vi "filter.get.state.vi"(11 "filter.data in":T1 {"get.state"."v"."Quantity" format="%.0x"; "get.state"."v"."OrderId" format="%.0x"; "mem.cmd"."ord.2"."v"."Quantity" format="%016x"; "mem.cmd"."ord.2"."v"."OrderId" format="%016x"; "mem.cmd"."ord.1"."v"."Quantity" format="%016x"; "mem.cmd"."ord.1"."v"."OrderId" format="%016x"; "mem.cmd"."ticker"."v"."Symbol" format="%016x"; "mem.cmd"."order.slot.value"."Quantity" format="%016x"; "mem.cmd"."order.slot.value"."OrderId" format="%016x"; "debug"."v"."slot.3" format="%.0x"; "debug"."v"."slot.2" format="%.0x"; "debug"."v"."slot.1" format="%.0x"; "debug"."v"."slot.0" format="%.0x"; "Scratch"."OrderId" format="%016x"; "hash.2"."data.in" format="%.0x"; "hash.2"."crc32.out" format="%.0x"; "hash.1"."data.in" format="%.0x"; "hash.1"."crc32.out" format="%.0x"}) -> (3 "filter.data out":T1 {"get.state"."v"."Quantity" format="%.0x"; "get.state"."v"."OrderId" format="%.0x"; "mem.cmd"."ord.2"."v"."Quantity" format="%016x"; "mem.cmd"."ord.2"."v"."OrderId" format="%016x"; "mem.cmd"."ord.1"."v"."Quantity" format="%016x"; "mem.cmd"."ord.1"."v"."OrderId" format="%016x"; "mem.cmd"."ticker"."v"."Symbol" format="%016x"; "mem.cmd"."order.slot.value"."Quantity" format="%016x"; "mem.cmd"."order.slot.value"."OrderId" format="%016x"; "debug"."v"."slot.3" format="%.0x"; "debug"."v"."slot.2" format="%.0x"; "debug"."v"."slot.1" format="%.0x"; "debug"."v"."slot.0" format="%.0x"; "Scratch"."OrderId" format="%016x"; "hash.2"."data.in" format="%.0x"; "hash.2"."crc32.out" format="%.0x"; "hash.1"."data.in" format="%.0x"; "hash.1"."crc32.out" format="%.0x"})   [LabVIEW 2020]
uses:
  order.slot.ctl
  ticker.slot.ctl
  filter.memory.command.ctl
  filter.states.ctl
  filter.state.slot.ctl
  filter.state.ctl
  order.slot.hm.ctl
  order.slot.access.ctl
  ticker.slot.access.ctl
  filter.debug.slot.ctl
  filter.debug.ctl
  filter.data.scratch.ctl
  Market.Data.Common/fpga/orderbook.command.ctl
  Market.Data.Common/fpga/fpganow.common.fpga.lvlib
  filter.data.ctl
  Market.Data.Common/fpga/orderbook.command.type.ctl
  filter.hash.ctl
  Filter.lvclass
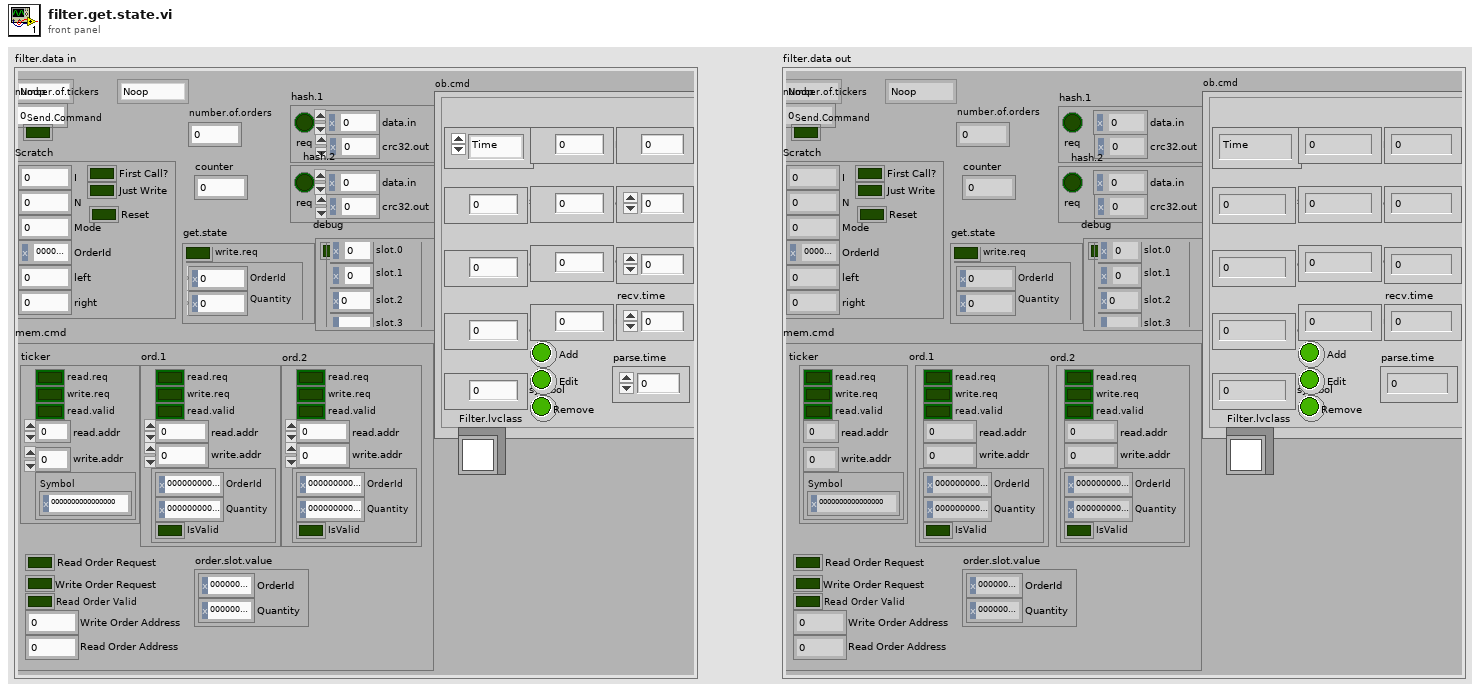
[diagram p1: front panel]
types:
  T1 = typedef "filter.data.ctl" = cluster{"filter.state":T2, "number.of.tickers":u32, "filter.saved.state":T2, "Send.Command":bool, "hash.1":T3, "hash.2":T3, "Scratch":T4, "debug":T5, "mem.cmd":T7, "get.state":T13, "ob.cmd":T15, "number.of.orders":u32, "Filter.lvclass":refnum<class "Filter.lvclass">, "counter":i16}
  T2 = typedef "filter.states.ctl" = enum16{"Noop", "Reset", "Debug", "Configuration", "Wait.for.Command", "Filter.Add", "Filter.Other", "Insert.Order", "Delete Order", "Get.State", "Get.Watchlist", "Get.Memory"}
  T3 = typedef "filter.hash.ctl" = cluster{"req":bool, "data.in":u64, "crc32.out":u32}
  T4 = typedef "filter.data.scratch.ctl" = cluster{"I":u32, "N":u32, "Mode":u32, "OrderId":u64, "First Call?":bool, "Just Write":bool, "left":u32, "right":u32, "Reset":bool}
  T5 = typedef "filter.debug.ctl" = cluster{"write":bool, "v":T6}
  T6 = typedef "filter.debug.slot.ctl" = cluster{"slot.0":u64, "slot.1":u64, "slot.2":u64, "slot.3":u64}
  T7 = typedef "filter.memory.command.ctl" = cluster{"Read Order Request":bool, "Write Order Request":bool, "Read Order Valid":bool, "Write Order Address":u32, "Read Order Address":u32, "order.slot.value":T8, "ticker":T9, "ord.1":T11, "ord.2":T11}
  T8 = typedef "order.slot.ctl" = cluster{"OrderId":u64, "Quantity":u64}
  T9 = typedef "ticker.slot.access.ctl" = cluster{"read.req":bool, "write.req":bool, "read.valid":bool, "read.addr":u32, "write.addr":u32, "v":T10}
  T10 = typedef "ticker.slot.ctl" = cluster{"Symbol":u64}
  T11 = typedef "order.slot.access.ctl" = cluster{"read.req":bool, "write.req":bool, "read.valid":bool, "read.addr":u32, "write.addr":u32, "v":T12}
  T12 = typedef "order.slot.hm.ctl" = cluster{"OrderId":u64, "Quantity":u64, "IsValid":bool}
  T13 = typedef "filter.state.ctl" = cluster{"write.req":bool, "v":T14}
  T14 = typedef "filter.state.slot.ctl" = cluster{"OrderId":u64, "Quantity":u64}
  T15 = typedef "fpganow.common.fpga.lvlib/orderbook.command.ctl" = cluster{"type":T16, "side":u8, "orderId ":u64, "quantity":u32, "symbol":u64, "price":u64, "executed.qty":u32, "canceled.qty":u32, "remaining.qty":u32, "seconds":u64, "nanoseconds":u64, "Add":bool, "Edit":bool, "Remove":bool, "seq no":u32, "recv.time":u64, "parse.time":u64}
  T16 = typedef "fpganow.common.fpga.lvlib/orderbook.command.type.ctl" = enum8{"Time", "AddOrder", "OrderExecuted", "OrderExecutedAtPrice", "ReduceSize", "ModifyOrder", "DeleteOrder", "Get.Everything", "Get.All.Orders", "Get.Top"}
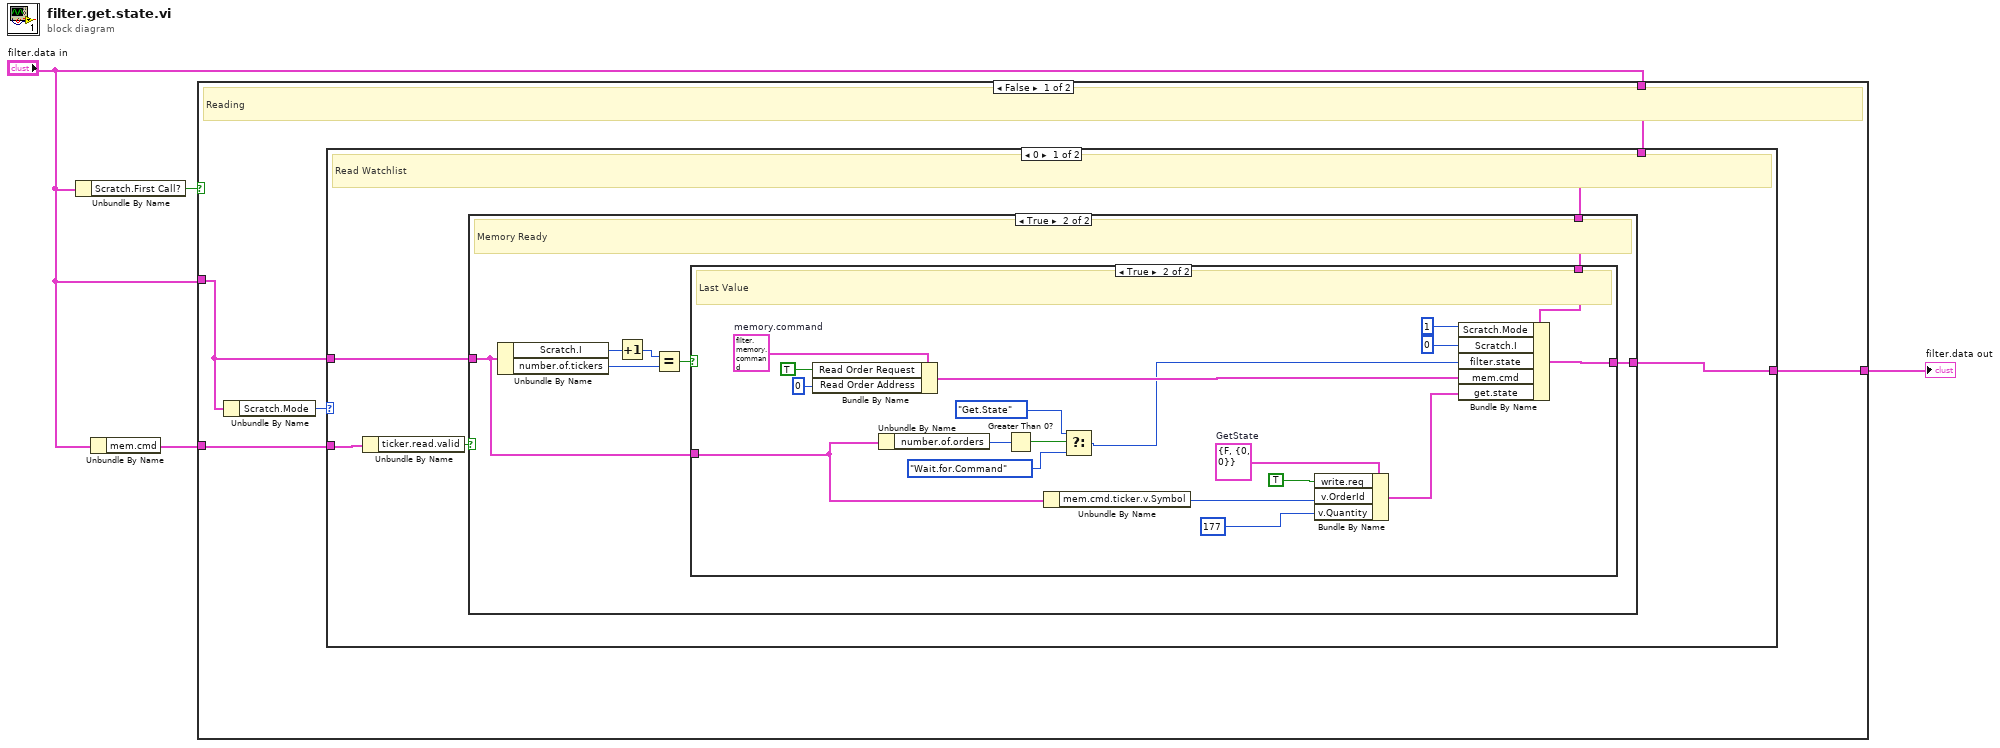
[diagram p0: block diagram]
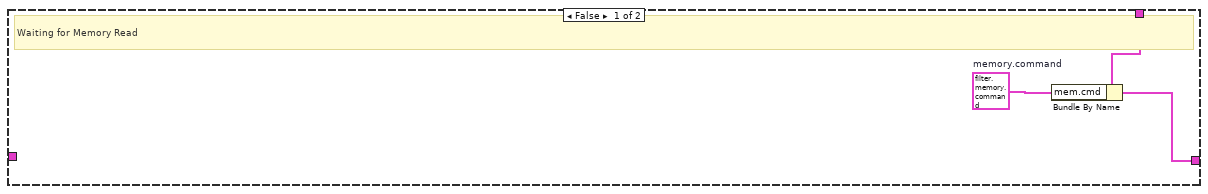
[diagram p2: hidden frame]
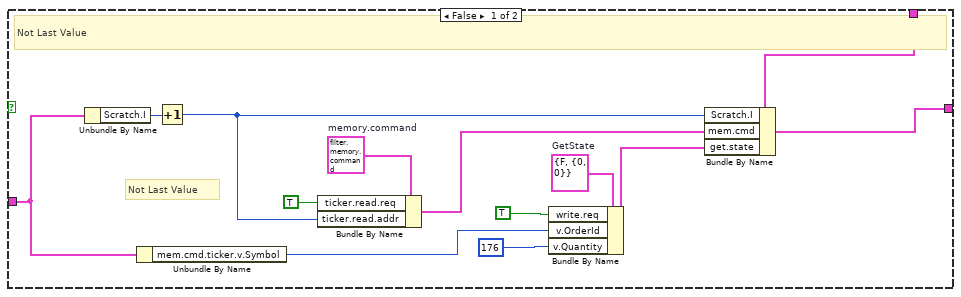
[diagram p3: hidden frame]
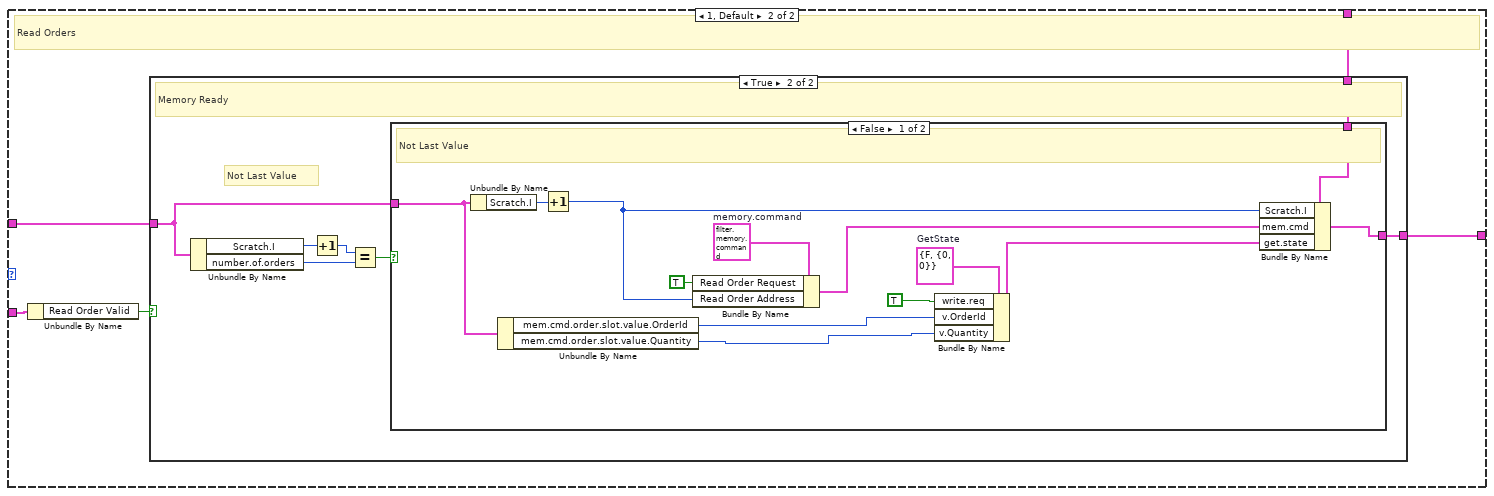
[diagram p4: hidden frame]
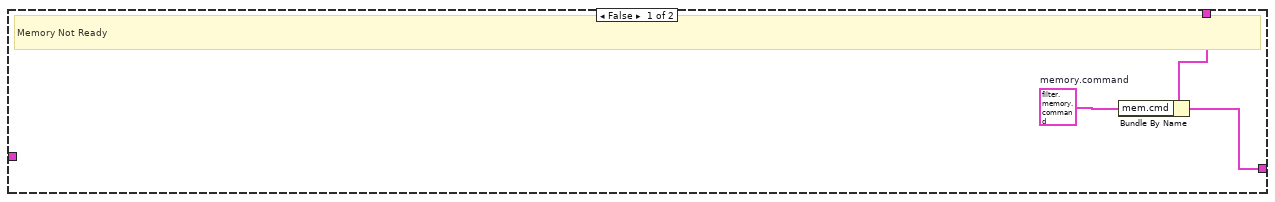
[diagram p5: hidden frame]
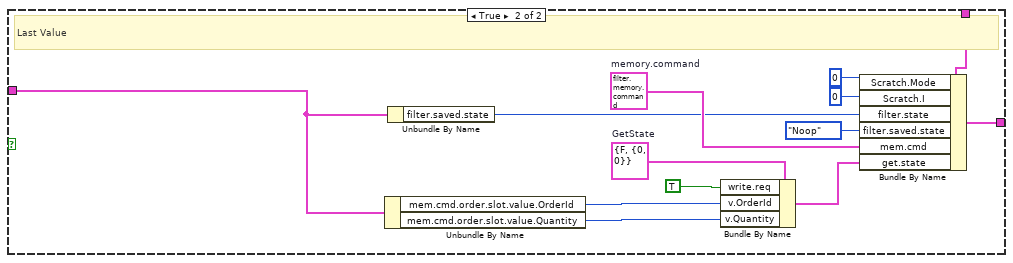
[diagram p6: hidden frame]
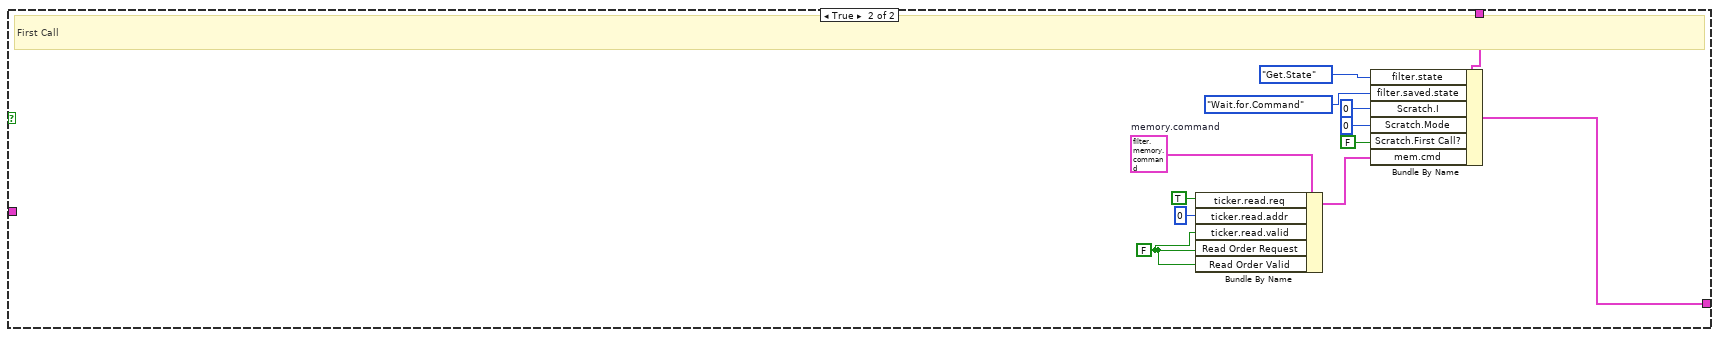
[diagram p7: hidden frame]
diagram:
  n1 = Unbundle By Name("filter.data in") -> ("Scratch.First Call?"=w1:bool)
  n2 = Unbundle By Name("filter.data in") -> ("mem.cmd"=w4:T7)
  n3 = case shown="False" w1 {
    tunnel: "filter.data in" -> [w8 w109]
    tunnel: [w9 w108] -> w2
    tunnel: "filter.data in" -> [w6 _]
    tunnel: w4 -> [w7 _]
    frame False {
      # "Reading"
      n4 = Unbundle By Name(w6) -> ("Scratch.Mode"=w5:u32)
      n5 = case shown="0" w5 {
        tunnel: [w14 w61] -> w9
        tunnel: w8 -> [w13 w60]
        tunnel: w7 -> [w11 w58]
        tunnel: w6 -> [w10 w57]
        frame 0 {
          # "Read Watchlist"
          n6 = Unbundle By Name(w11) -> ("ticker.read.valid"=w12:bool)
          n7 = case shown="True" w12 {
            tunnel: [w15 w18] -> w14
            tunnel: w13 -> [w17 w19]
            tunnel: w10 -> [_ w20]
            frame False {
              w16 = T7 {"Read Order Request"=FALSE, "Write Order Request"=FALSE, "Read Order Valid"=FALSE, "Write Order Address"=0, "Read Order Address"=0, "order.slot.value"={"OrderId"=0, "Quantity"=0}, "ticker"={"read.req"=FALSE, "write.req"=FALSE, "read.valid"=FALSE, "read.addr"=0, "write.addr"=0, "v"={"Symbol"=0}}, "ord.1"={"read.req"=FALSE, "write.req"=FALSE, "read.valid"=FALSE, "read.addr"=0, "write.addr"=0, "v"={"OrderId"=0, "Quantity"=0, "IsValid"=FALSE}}, "ord.2"={"read.req"=FALSE, "write.req"=FALSE, "read.valid"=FALSE, "read.addr"=0, "write.addr"=0, "v"={"OrderId"=0, "Quantity"=0, "IsValid"=FALSE}}}  # memory.command
              # "Waiting for Memory Read"
              n8 = Bundle By Name(cluster=w17, "mem.cmd"=w16) -> (w15:T1)
            }
            frame True {
              # "Memory Ready"
              n9 = Unbundle By Name(w20) -> ("Scratch.I"=w24:u32, "number.of.tickers"=w22:u32)
              n10 = Increment(x=w24) -> (x+1=w23:u32)
              n11 = Equal?(x=w23, y=w22) -> (x = y?=w21:bool)
              n12 = case shown="True" w21 {
                tunnel: w20 -> [w30 w43]
                tunnel: w19 -> [w26 w56]
                tunnel: [w37 w55] -> w18
                frame False {
                  w33 = T13 {"write.req"=FALSE, "v"={"OrderId"=0, "Quantity"=0}}  # GetState
                  w36 = T7 {"Read Order Request"=FALSE, "Write Order Request"=FALSE, "Read Order Valid"=FALSE, "Write Order Address"=0, "Read Order Address"=0, "order.slot.value"={"OrderId"=0, "Quantity"=0}, "ticker"={"read.req"=FALSE, "write.req"=FALSE, "read.valid"=FALSE, "read.addr"=0, "write.addr"=0, "v"={"Symbol"=0}}, "ord.1"={"read.req"=FALSE, "write.req"=FALSE, "read.valid"=FALSE, "read.addr"=0, "write.addr"=0, "v"={"OrderId"=0, "Quantity"=0, "IsValid"=FALSE}}, "ord.2"={"read.req"=FALSE, "write.req"=FALSE, "read.valid"=FALSE, "read.addr"=0, "write.addr"=0, "v"={"OrderId"=0, "Quantity"=0, "IsValid"=FALSE}}}  # memory.command
                  # "Not Last Value"
                  # "Not Last Value"
                  n13 = Unbundle By Name(w30) -> ("Scratch.I"=w34:u32)
                  n14 = Unbundle By Name(w30) -> ("mem.cmd.ticker.v.Symbol"=w29:u64)
                  n15 = Increment(x=w34) -> (x+1=w27:u32)
                  n16 = Bundle By Name(cluster=w36, "ticker.read.req"=TRUE ("Read.Request"), "ticker.read.addr"=w27) -> (w35:T7)
                  n17 = Bundle By Name(cluster=w33, "write.req"=TRUE ("Write.to.Debug"), "v.OrderId"=w29, "v.Quantity"=u64 176 ("debug.slot.OrderId")) -> (w32:T13)
                  n18 = Bundle By Name(cluster=w26, "Scratch.I"=w27, "mem.cmd"=w35, "get.state"=w32) -> (w37:T1)
                }
                frame True {
                  w44 = T13 {"write.req"=FALSE, "v"={"OrderId"=0, "Quantity"=0}}  # GetState
                  w48 = T7 {"Read Order Request"=FALSE, "Write Order Request"=FALSE, "Read Order Valid"=FALSE, "Write Order Address"=0, "Read Order Address"=0, "order.slot.value"={"OrderId"=0, "Quantity"=0}, "ticker"={"read.req"=FALSE, "write.req"=FALSE, "read.valid"=FALSE, "read.addr"=0, "write.addr"=0, "v"={"Symbol"=0}}, "ord.1"={"read.req"=FALSE, "write.req"=FALSE, "read.valid"=FALSE, "read.addr"=0, "write.addr"=0, "v"={"OrderId"=0, "Quantity"=0, "IsValid"=FALSE}}, "ord.2"={"read.req"=FALSE, "write.req"=FALSE, "read.valid"=FALSE, "read.addr"=0, "write.addr"=0, "v"={"OrderId"=0, "Quantity"=0, "IsValid"=FALSE}}}  # memory.command
                  # "Last Value"
                  n19 = Bundle By Name(cluster=w48, "Read Order Request"=TRUE ("Read Order\nRequest"), "Read Order Address"=u32 0 ("Read Order\nAddress")) -> (w47:T7)
                  n20 = Unbundle By Name(w43) -> ("number.of.orders"=w42:u32)
                  n21 = Greater Than 0?(x=w42) -> (x > 0?=w41:bool)
                  n22 = Unbundle By Name(w43) -> ("mem.cmd.ticker.v.Symbol"=w52:u64)
                  n23 = Select(t=filter.states."Get.State" ("filter.state"), s=w41, f=filter.states."Wait.for.Command") -> (s? t:f=w39:T2)
                  n24 = Bundle By Name(cluster=w44, "write.req"=TRUE ("Write.to.Debug"), "v.OrderId"=w52, "v.Quantity"=u64 177 ("debug.slot.OrderId")) -> (w54:T13)
                  n25 = Bundle By Name(cluster=w56, "Scratch.Mode"=u32 1, "Scratch.I"=u32 0, "filter.state"=w39, "mem.cmd"=w47, "get.state"=w54) -> (w55:T1)
                }
              }
            }
          }
        }
        frame 1, Default {
          # "Read Orders"
          n26 = Unbundle By Name(w58) -> ("Read Order Valid"=w59:bool)
          n27 = case shown="True" w59 {
            tunnel: [w62 w65] -> w61
            tunnel: w60 -> [w64 w66]
            tunnel: w57 -> [_ w67]
            frame False {
              w63 = T7 {"Read Order Request"=FALSE, "Write Order Request"=FALSE, "Read Order Valid"=FALSE, "Write Order Address"=0, "Read Order Address"=0, "order.slot.value"={"OrderId"=0, "Quantity"=0}, "ticker"={"read.req"=FALSE, "write.req"=FALSE, "read.valid"=FALSE, "read.addr"=0, "write.addr"=0, "v"={"Symbol"=0}}, "ord.1"={"read.req"=FALSE, "write.req"=FALSE, "read.valid"=FALSE, "read.addr"=0, "write.addr"=0, "v"={"OrderId"=0, "Quantity"=0, "IsValid"=FALSE}}, "ord.2"={"read.req"=FALSE, "write.req"=FALSE, "read.valid"=FALSE, "read.addr"=0, "write.addr"=0, "v"={"OrderId"=0, "Quantity"=0, "IsValid"=FALSE}}}  # memory.command
              # "Memory Not Ready"
              n28 = Bundle By Name(cluster=w64, "mem.cmd"=w63) -> (w62:T1)
            }
            frame True {
              # "Not Last Value"
              # "Memory Ready"
              n29 = Unbundle By Name(w67) -> ("Scratch.I"=w71:u32, "number.of.orders"=w69:u32)
              n30 = Increment(x=w71) -> (x+1=w70:u32)
              n31 = Equal?(x=w70, y=w69) -> (x = y?=w68:bool)
              n32 = case shown="False" w68 {
                tunnel: w67 -> [w78 w93]
                tunnel: w66 -> [w76 w97]
                tunnel: [w84 w96] -> w65
                frame False {
                  w72 = T13 {"write.req"=FALSE, "v"={"OrderId"=0, "Quantity"=0}}  # GetState
                  w83 = T7 {"Read Order Request"=FALSE, "Write Order Request"=FALSE, "Read Order Valid"=FALSE, "Write Order Address"=0, "Read Order Address"=0, "order.slot.value"={"OrderId"=0, "Quantity"=0}, "ticker"={"read.req"=FALSE, "write.req"=FALSE, "read.valid"=FALSE, "read.addr"=0, "write.addr"=0, "v"={"Symbol"=0}}, "ord.1"={"read.req"=FALSE, "write.req"=FALSE, "read.valid"=FALSE, "read.addr"=0, "write.addr"=0, "v"={"OrderId"=0, "Quantity"=0, "IsValid"=FALSE}}, "ord.2"={"read.req"=FALSE, "write.req"=FALSE, "read.valid"=FALSE, "read.addr"=0, "write.addr"=0, "v"={"OrderId"=0, "Quantity"=0, "IsValid"=FALSE}}}  # memory.command
                  # "Not Last Value"
                  n33 = Unbundle By Name(w78) -> ("Scratch.I"=w81:u32)
                  n34 = Unbundle By Name(w78) -> ("mem.cmd.order.slot.value.OrderId"=w73:u64, "mem.cmd.order.slot.value.Quantity"=w74:u64)
                  n35 = Increment(x=w81) -> (x+1=w75:u32)
                  n36 = Bundle By Name(cluster=w83, "Read Order Request"=TRUE ("Read.Request"), "Read Order Address"=w75) -> (w82:T7)
                  n37 = Bundle By Name(cluster=w72, "write.req"=TRUE ("Write.to.Debug"), "v.OrderId"=w73, "v.Quantity"=w74) -> (w80:T13)
                  n38 = Bundle By Name(cluster=w76, "Scratch.I"=w75, "mem.cmd"=w82, "get.state"=w80) -> (w84:T1)
                }
                frame True {
                  w85 = T13 {"write.req"=FALSE, "v"={"OrderId"=0, "Quantity"=0}}  # GetState
                  w92 = T7 {"Read Order Request"=FALSE, "Write Order Request"=FALSE, "Read Order Valid"=FALSE, "Write Order Address"=0, "Read Order Address"=0, "order.slot.value"={"OrderId"=0, "Quantity"=0}, "ticker"={"read.req"=FALSE, "write.req"=FALSE, "read.valid"=FALSE, "read.addr"=0, "write.addr"=0, "v"={"Symbol"=0}}, "ord.1"={"read.req"=FALSE, "write.req"=FALSE, "read.valid"=FALSE, "read.addr"=0, "write.addr"=0, "v"={"OrderId"=0, "Quantity"=0, "IsValid"=FALSE}}, "ord.2"={"read.req"=FALSE, "write.req"=FALSE, "read.valid"=FALSE, "read.addr"=0, "write.addr"=0, "v"={"OrderId"=0, "Quantity"=0, "IsValid"=FALSE}}}  # memory.command
                  # "Last Value"
                  n39 = Unbundle By Name(w93) -> ("mem.cmd.order.slot.value.OrderId"=w87:u64, "mem.cmd.order.slot.value.Quantity"=w86:u64)
                  n40 = Unbundle By Name(w93) -> ("filter.saved.state"=w91:T2)
                  n41 = Bundle By Name(cluster=w85, "write.req"=TRUE ("Write.to.Debug"), "v.OrderId"=w87, "v.Quantity"=w86) -> (w95:T13)
                  n42 = Bundle By Name(cluster=w97, "Scratch.Mode"=u32 0, "Scratch.I"=u32 0, "filter.state"=w91, "filter.saved.state"=filter.states."Noop", "mem.cmd"=w92, "get.state"=w95) -> (w96:T1)
                }
              }
            }
          }
        }
      }
    }
    frame True {
      w99 = FALSE ("Read Ticker Valid")
      w104 = T7 {"Read Order Request"=FALSE, "Write Order Request"=FALSE, "Read Order Valid"=FALSE, "Write Order Address"=0, "Read Order Address"=0, "order.slot.value"={"OrderId"=0, "Quantity"=0}, "ticker"={"read.req"=FALSE, "write.req"=FALSE, "read.valid"=FALSE, "read.addr"=0, "write.addr"=0, "v"={"Symbol"=0}}, "ord.1"={"read.req"=FALSE, "write.req"=FALSE, "read.valid"=FALSE, "read.addr"=0, "write.addr"=0, "v"={"OrderId"=0, "Quantity"=0, "IsValid"=FALSE}}, "ord.2"={"read.req"=FALSE, "write.req"=FALSE, "read.valid"=FALSE, "read.addr"=0, "write.addr"=0, "v"={"OrderId"=0, "Quantity"=0, "IsValid"=FALSE}}}  # memory.command
      # "First Call"
      n43 = Bundle By Name(cluster=w104, "ticker.read.req"=TRUE ("Read Ticker\nRequest"), "ticker.read.addr"=u32 0 ("Read Ticker\nAddress"), "ticker.read.valid"=w99, "Read Order Request"=w99, "Read Order Valid"=w99) -> (w101:T7)
      n44 = Bundle By Name(cluster=w109, "filter.state"=filter.states."Get.State", "filter.saved.state"=filter.states."Wait.for.Command", "Scratch.I"=u32 0, "Scratch.Mode"=u32 0, "Scratch.First Call?"=FALSE, "mem.cmd"=w101) -> (w108:T1)
    }
  }
  "filter.data out" <- w2
